vi "Set Scaling Factor.vi"(8 "error in (no error)":errorcluster, 10 "Value":dbl, 11 "QR Code Detector in":refnum<class "QR Code Detector.lvclass">) -> (0 "error out":errorcluster, 3 "QR Code Detector (Duplicate)":refnum<class "QR Code Detector.lvclass">)   [LabVIEW 2020, in "feature_detection.lvlib" / "QR Code Detector.lvclass"]
uses:
  QR Code Detector.lvclass
  QR Code Detector.lvclass/QR Code Detector.ctl
  common/Module Path.vi
  <vilib>/Utility/error.llb/Error Cluster From Error Code.vi
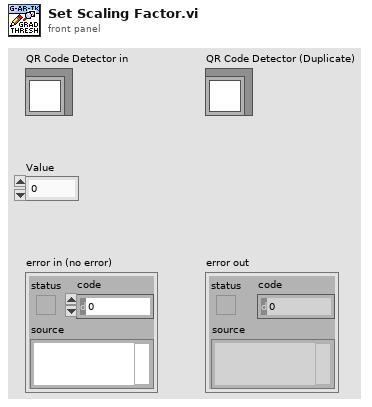
[diagram p1: front panel]
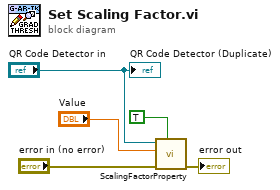
[diagram p0: block diagram]
diagram:
  n1 = call "ScalingFactorProperty.vi"("Write?"=TRUE, "error in (no error)"="error in (no error)", "Value in"="Value", "QR Code Detector in"="QR Code Detector in") -> ("error out"=→"error out":errorcluster)  [unwired: 6 in, 1 out]
  "QR Code Detector (Duplicate)" <- "QR Code Detector in"
